vi "Axis Camera_2012.vi"() -> ()   [LabVIEW 2012]
panel:
  in  "URL of Camera":string="http://cameras ip address"
  in  "stop":bool
  in  "Load browser":bool
  out "Title":string
  in  "WebBrowser":refnum<k7>(container)
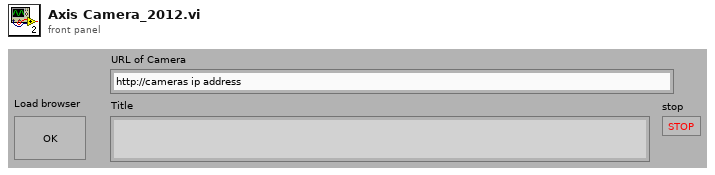
[diagram p1: front panel]
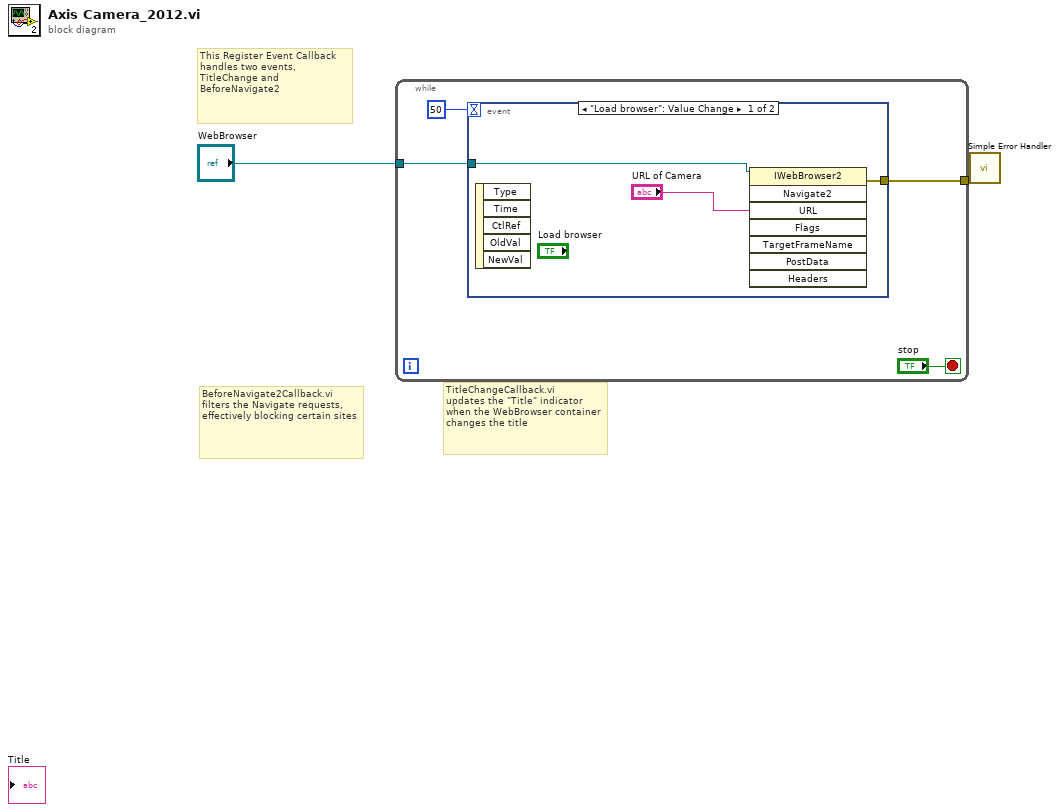
[diagram p0: block diagram]
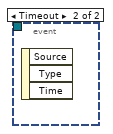
[diagram p2: hidden frame]
diagram:
  # "TitleChangeCallback.vi\nupdates the \"Title\" indicator when the WebBrowser container changes the title"
  # "BeforeNavigate2Callback.vi\nfilters the Navigate requests,\neffectively blocking certain sites"
  # "This Register Event Callback\nhandles two events, TitleChange and BeforeNavigate2"
  n1 = while {
    tunnel: "WebBrowser" -> [w6]
    tunnel: [w4] -> w1
    stop <- "stop" stop-if-true
    n2 = event shown="[0] \"Load browser\": Value Change" {
      selector: _ -> [_ _]
      dyn-events: _ -> [_ _]
      timeout: 50 -> [_ _]
      tunnel: w6 -> [w9 _]
      tunnel: [w7 _] -> w4
      event "Load browser": Value Change {
        n3 = event-data() -> ()  [unwired: 6 out]
        n4 = invoke class="IWebBrowser2" method="Navigate2"(reference=w9, "URL"="URL of Camera") -> (error out=w7:errorcluster)  [unwired: 6 in, 7 out]
      }
      event Timeout {
        n5 = event-data() -> ()  [unwired: 4 out]
      }
    }
  }
  n6 = call <vilib>:"Simple Error Handler.vi"("error in (no error)"=w1) -> ()  [unwired: 1 in, 8 out]
